vi "IndexCheckifBelow0_171213.vi"   [LabVIEW 2016]
uses:
  Globaltracker.vi
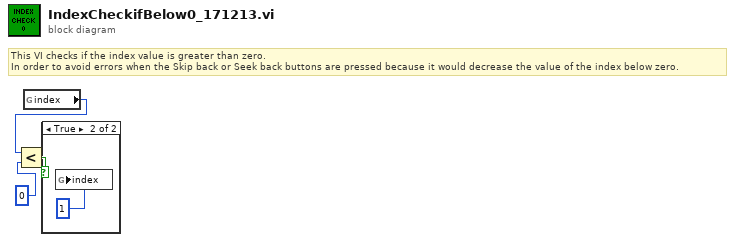
[diagram p0: block diagram]
diagram:
  # "This VI checks if the index value is greater than zero.\nIn order to avoid errors when the Skip back or Seek back buttons are pressed because it would decrease the value of the index below zero."
  n1 = global read "Globaltracker.vi" "index"() -> (w3:i16)
  n2 = Less?(x=w3, y=0) -> (x < y?=w1:bool)
  n3 = case shown="True" w1 {
    frame False {
    }
    frame True {
      n4 = global write "Globaltracker.vi" "index"(1 ("index")) -> ()
    }
  }
